vi "TDK_CloseCom.vi"(11 "VISA name":refnum<visa-resource-name>) -> (0 "error out (no error)":errorcluster)   [LabVIEW 2015]
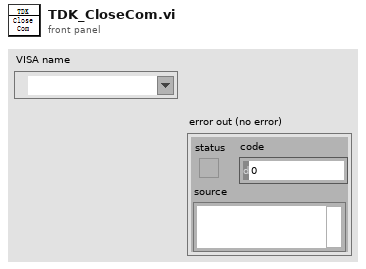
[diagram p1: front panel]
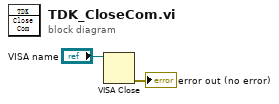
[diagram p0: block diagram]
diagram:
  n1 = VISA Close(VISA resource name="VISA name") -> (error out=→"error out (no error)":errorcluster)  [unwired: 1 in]
